vi "Action Name.vi"(11 "AddProjAction in":refnum<class "AddProjAction.lvclass">) -> (2 "Action Name":string)   [LabVIEW 2020, in "AddProjAction.lvclass"]
uses:
  AddProjAction.lvclass
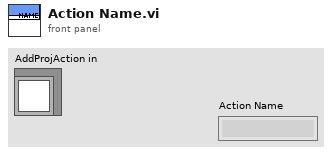
[diagram p1: front panel]
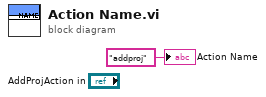
[diagram p0: block diagram]
diagram:
  "Action Name" <- "addproj" ("Action Name")
